vi "GV_YscaleDrawPicture.vi"(9 "Yscale properties":T1={"X-position"=150, "top"=40, "bottom"=200, "max range"=100.0, "min range"=0.0, "color"=255, "Plot bottom"=50, "TagName"=""}, 11 "Picture IN":picture) -> (3 "Picture OUT":picture)   [LabVIEW 2020, in "Sgraph_lib_V1.lvlib" / "Gviewer.lvclass"]
doc: "Andre Koelewijn, 12 sept 2014 Rev 0\nThis vi draws an Y-axis scale to plot within the plot area of a graph.\nThe subvi's used are modified vi's from the NI library in such a way that they\nmeet proper Y-axis scale indication for the historian graph."
uses:
  Gviewer.lvclass
  controls/Typedef_YscaleProp.ctl
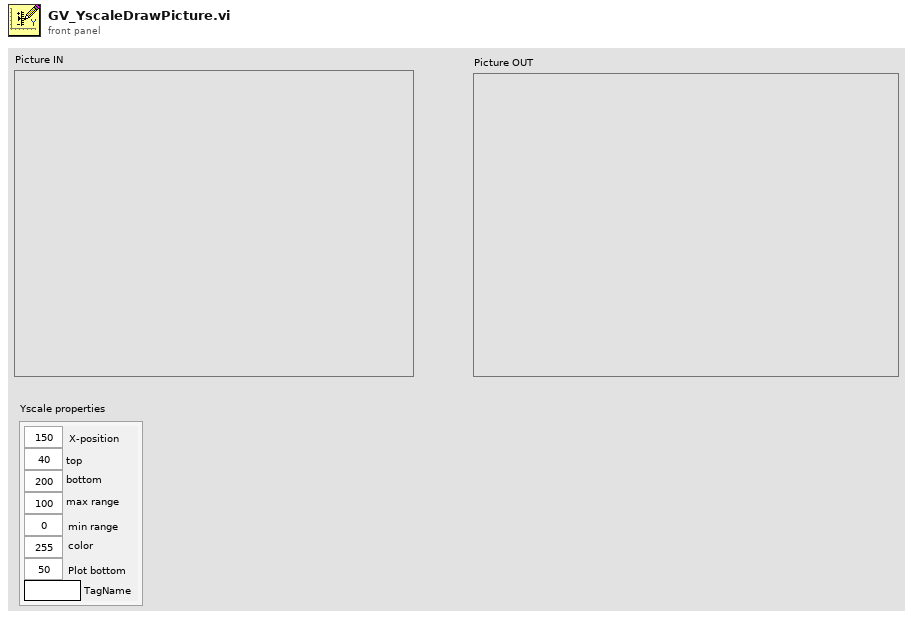
[diagram p1: front panel]
types:
  T1 = typedef "Typedef_YscaleProp.ctl" = cluster{"X-position":i16, "top":i16, "bottom":i16, "max range":dbl, "min range":dbl, "color":u32, "Plot bottom":i16, "TagName":string}
  T2 = cluster{"coordinate 1":i16, "value 1":dbl, "coordinate 2":i16, "value 2":dbl, "log?(F)":bool}
  T3 = cluster{"horizontal":bool, "left/top":bool, "draw bar":bool, "line color":u32, "text color(black)":u32}
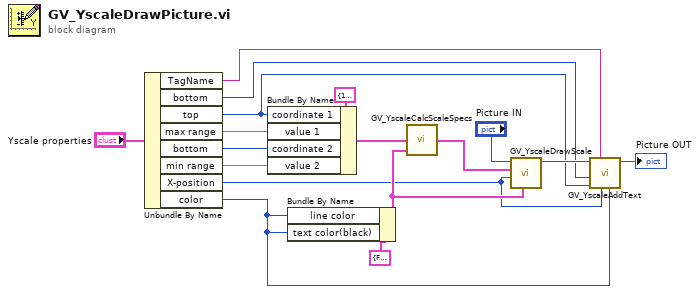
[diagram p0: block diagram]
diagram:
  n1 = Unbundle By Name("Yscale properties") -> ("TagName"=w3:string, "bottom"=w5:i16, "top"=w4:i16, "max range"=w12:dbl, "bottom"=w11:i16, "min range"=w10:dbl, "X-position"=w1:i16, "color"=w2:u32)
  n2 = Bundle By Name(cluster=T2 {"coordinate 1"=10, "value 1"=30.0, "coordinate 2"=400, "value 2"=0.0, "log?(F)"=FALSE} ("scale definition"), "coordinate 1"=w4, "value 1"=w12, "coordinate 2"=w11, "value 2"=w10) -> (w15:T2)
  n3 = Bundle By Name(cluster=T3 {"horizontal"=FALSE, "left/top"=FALSE, "draw bar"=TRUE, "line color"=0, "text color(black)"=0} ("scale attributes"), "line color"=w2, "text color(black)"=w2) -> (w8:T3)
  n4 = call "GV_YscaleCalcScaleSpecs.vi"("scale definition"=w15, "scale attributes"=w8) -> ("scale specs"=w17:cluster{"coordinate":i16, "label":string}[])  [unwired: 7 in]
  n5 = call "GV_YscaleDrawScale.vi"("scale attributes"=w8, "constant coordinate"=w1, "scale specs"=w17, "picture"="Picture IN") -> ("new picture"=w7:picture)  [unwired: 7 in]
  n6 = call "GV_YscaleAddText.vi"("Color"=w2, "X-position"=w1, "Tagname"=w3, "Scale top"=w4, "Plot bottom"=w5, "2D Picture IN"=w7) -> ("2D Picture OUT"=→"Picture OUT":picture)  [unwired: 5 in]
